vi "RunTest.vi"(8 "error in (no error)":errorcluster, 11 "Fact in":refnum<class "Fact.lvclass">) -> (0 "error out":errorcluster, 3 "Fact out":refnum<class "Fact.lvclass">)   [LabVIEW 2019, in "TestCase.lvlib" / "Fact.lvclass"]
doc: "Override to run the test and assert its state."
uses:
  Fact.lvclass
  Fact.lvclass/Fact.ctl
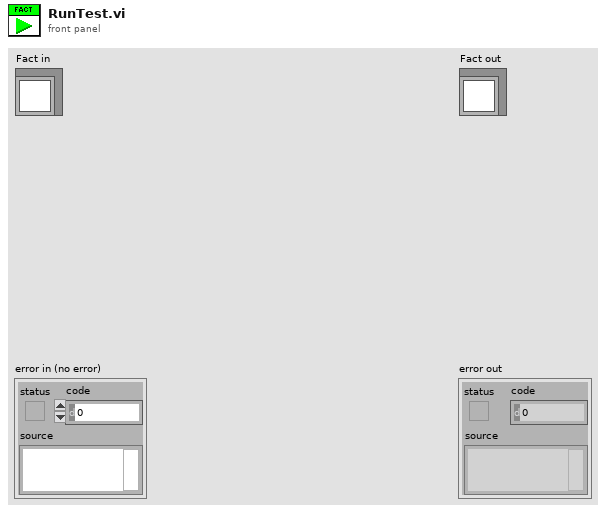
[diagram p1: front panel]
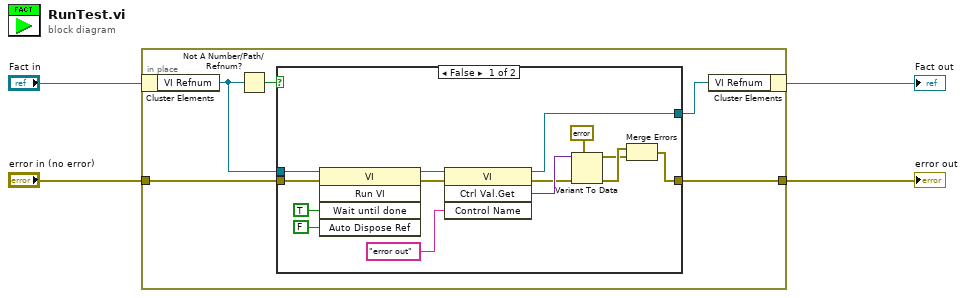
[diagram p0: block diagram]
diagram:
  n1 = in-place {
    in-place-border: "error in (no error)" -> [w8]
    in-place-border: [w7] -> w2
    n2 = in-place-cluster #1("Fact in") -> ("VI Refnum"=w6:refnum<vi>)
    n3 = Not A Number/Path/Refnum?(number/path/refnum=w6) -> (NaN/Path/Refnum?=w5:bool)
    n4 = case shown="False" w5 {
      tunnel: [w15 w25] -> w9
      tunnel: w8 -> [w14 w24]
      tunnel: [w13 w24] -> w7
      tunnel: w6 -> [w11 w25]
      frame False {
        n5 = invoke class="VI" method="Run VI"(reference=w11, error in=w14, "Wait until done"=TRUE ("Wait Until Done"), "Auto Dispose Ref"=FALSE ("Auto Dispose Reference")) -> (reference out=w20:refnum<vi>, error out=w19:errorcluster)  [unwired: 1 in, 3 out]
        n6 = invoke class="VI" method="Ctrl Val.Get"(reference=w20, error in=w19, "Control Name"="error out") -> (reference out=w15:refnum<vi>, error out=w10:errorcluster, "Get Control Value Variant"=w17:variant)  [unwired: 1 in, 1 out]
        n7 = Variant To Data(error in=w10, type=errorcluster {"status"=FALSE, "code"=0, "source"=""}, Variant=w17) -> (data=w12:errorcluster, error out=w18:errorcluster)
        n8 = Merge Errors(w18, w12) -> (w13:errorcluster)
      }
      frame True {
      }
    }
    n9 = in-place-cluster #1("VI Refnum"=w9) -> (→"Fact out":refnum<class "Fact.lvclass">)
  }
  "error out" <- w2
